vi "Parse State with Arguments String.vi"(2 "State With Arguments":string="state >> arguments -> Callee") -> (6 "State":string="state", 7 "Arguments":string="arguments", 9 "Target Module":string="Callee", 10 "Message Symbol":string=" -> ")   [LabVIEW 2017, in "Communicable State Machine.lvlib"]
doc: "### Parse State with Arguments String.vi\n\n-- <b>Controls</b> --\n- <b>State with Arguments</b>:\nThe State string that requires the argument.\n\n-- <b>Indicators</b> --\n- <b>State</b>:\n- <b>Arguments</b>:\n- <b>Target Module</b>:\n- <b>Message Symbol</b>:"
uses:
  Communicable State Machine.lvlib
  <vilib>/regexp/Match Regular Expression.xnode
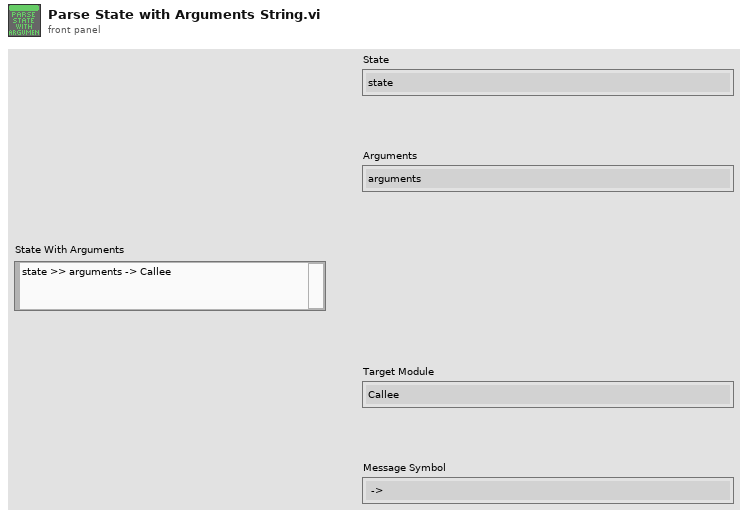
[diagram p1: front panel]
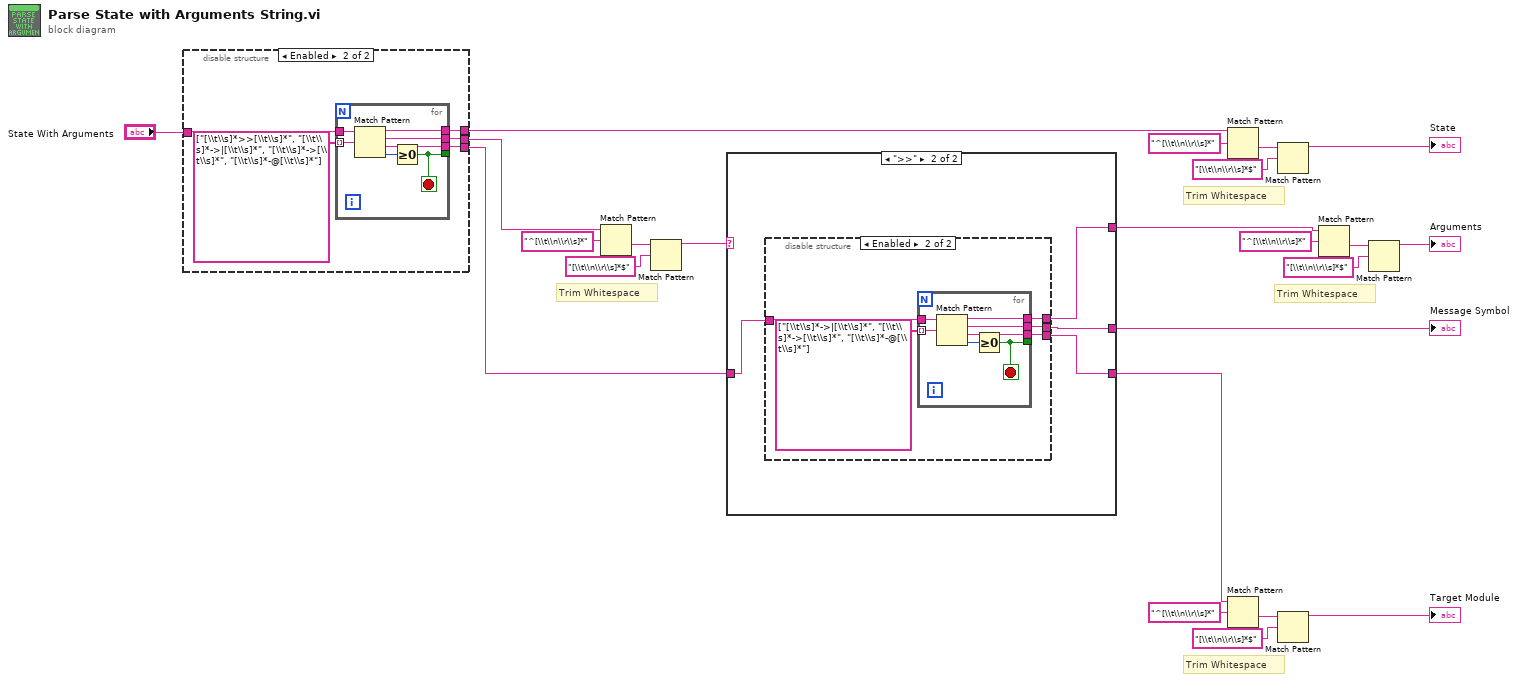
[diagram p0: block diagram]
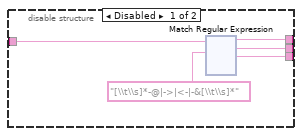
[diagram p3: hidden frame]
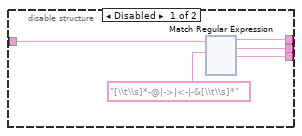
[diagram p4: hidden frame]
diagram:
  # "Trim Whitespace"
  # "Trim Whitespace"
  # "Trim Whitespace"
  # "Trim Whitespace"
  n1 = disable-structure shown="Enabled" {
    disable-tunnel: [w27 w145] -> w20
    disable-tunnel: [w26 w144] -> w10
    disable-tunnel: [w25 w143] -> w8
    disable-tunnel: "State With Arguments" -> [w24 w147]
    frame Disabled {
      n2 = xnode "Match Regular Expression"("input string"=w24, "regular expression"="[\\t\\s]*-@|->|<-|-&[\\t\\s]*") -> ("before match"=w27:string, "whole match"=w26:string, "after match"=w25:string)  [unwired: 4 in, 2 out]
    }
    frame Enabled {
      n3 = for {
        tunnel: w147 -> [w154]
        tunnel: string[] ["[\\t\\s]*>>[\\t\\s]*", "[\\t\\s]*->|[\\t\\s]*", "[\\t\\s]*->[\\t\\s]*", "[\\t\\s]*-@[\\t\\s]*"] -> [w153] mode=indexing
        tunnel: [w151] -> _
        tunnel: [w150] -> w145
        tunnel: [w149] -> w144
        tunnel: [w148] -> w143
        stop <- w151 stop-if-true
        n4 = Match Pattern(string=w154, regular expression=w153) -> (before substring=w150:string, match substring=w149:string, after substring=w148:string, offset past match=w152:i32)  [unwired: 1 in]
        n5 = Greater Or Equal To 0?(x=w152) -> (x >= 0?=w151:bool)
      }
    }
  }
  n6 = Match Pattern(string=w10, regular expression="^[\\t\\n\\r\\s]*") -> (after substring=w12:string)  [unwired: 1 in, 3 out]
  n7 = Match Pattern(string=w12, regular expression="[\\t\\n\\r\\s]*$") -> (before substring=w9:string)  [unwired: 1 in, 3 out]
  n8 = case shown="\">>\"" w9 {
    selector: w9 -> [w155 _]
    tunnel: w8 -> [w156 w160]
    tunnel: [w156 w157] -> w7
    tunnel: [w155 w159] -> w6
    tunnel: [_ w158] -> w1
    frame Default {
    }
    frame ">>" {
      n9 = disable-structure shown="Enabled" {
        disable-tunnel: [w164 w282] -> w158
        disable-tunnel: [w163 w281] -> w159
        disable-tunnel: [w162 w280] -> w157
        disable-tunnel: w160 -> [w161 w284]
        frame Disabled {
          n10 = xnode "Match Regular Expression"("input string"=w161, "regular expression"="[\\t\\s]*-@|->|<-|-&[\\t\\s]*") -> ("before match"=w164:string, "whole match"=w163:string, "after match"=w162:string)  [unwired: 4 in, 2 out]
        }
        frame Enabled {
          n11 = for {
            tunnel: w284 -> [w291]
            tunnel: string[] ["[\\t\\s]*->|[\\t\\s]*", "[\\t\\s]*->[\\t\\s]*", "[\\t\\s]*-@[\\t\\s]*"] -> [w290] mode=indexing
            tunnel: [w288] -> _
            tunnel: [w287] -> w282
            tunnel: [w286] -> w281
            tunnel: [w285] -> w280
            stop <- w288 stop-if-true
            n12 = Match Pattern(string=w291, regular expression=w290) -> (before substring=w287:string, match substring=w286:string, after substring=w285:string, offset past match=w289:i32)  [unwired: 1 in]
            n13 = Greater Or Equal To 0?(x=w289) -> (x >= 0?=w288:bool)
          }
        }
      }
    }
  }
  "Message Symbol" <- w6
  n14 = Match Pattern(string=w20, regular expression="^[\\t\\n\\r\\s]*") -> (after substring=w22:string)  [unwired: 1 in, 3 out]
  n15 = Match Pattern(string=w7, regular expression="^[\\t\\n\\r\\s]*") -> (after substring=w18:string)  [unwired: 1 in, 3 out]
  n16 = Match Pattern(string=w22, regular expression="[\\t\\n\\r\\s]*$") -> (before substring=→"State":string)  [unwired: 1 in, 3 out]
  n17 = Match Pattern(string=w18, regular expression="[\\t\\n\\r\\s]*$") -> (before substring=→"Target Module":string)  [unwired: 1 in, 3 out]
  n18 = Match Pattern(string=w1, regular expression="^[\\t\\n\\r\\s]*") -> (after substring=w3:string)  [unwired: 1 in, 3 out]
  n19 = Match Pattern(string=w3, regular expression="[\\t\\n\\r\\s]*$") -> (before substring=→"Arguments":string)  [unwired: 1 in, 3 out]
